vi "autoplace2.vi"(11 "Chain IN":bool) -> (3 "Chain OUT":bool)   [LabVIEW 2010, in "LASA Beta.lvrbt"]
uses:
  LASA Beta.lvrbt
  <vilib>/NXT/NXTIO Xnodes/AddressXNode/NXTIOAddress.xnode
  <vilib>/NXT/Subs/MotorXNode.Servo Type.ctl
  <vilib>/NXT/Subs/MotorXNode.1Servo.ctl
  <vilib>/NXT/Subs/LVHSConnector.ctl
  <vilib>/NXT/NXTIO Xnodes/NXTIOXNode/NXTIO.xnode
  op-run.vi
  <vilib>/NXT/Dual Mode Library/Waits/Wait_Num(msec).vi
  <vilib>/NXT/NXTIO Xnodes/NXTIONodeSubVIs/TETRIX IO Move Servos.vi
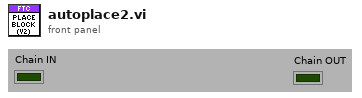
[diagram p1: front panel]
types:
  T1 = typedef "MotorXNode.Servo Type.ctl" = enum16{"Servo"}
  T2 = typedef "LVHSConnector.ctl" = cluster{"Hardware":string, "Flattened String":string}
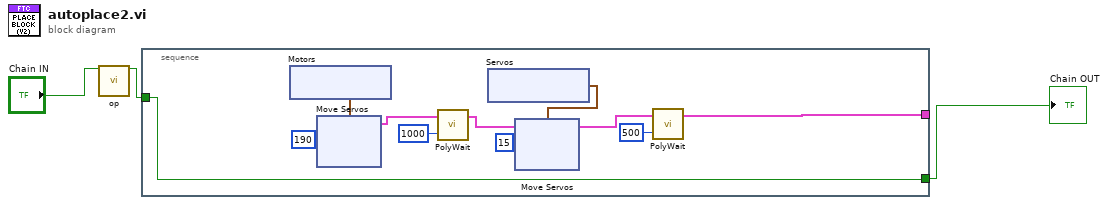
[diagram p0: block diagram]
diagram:
  n1 = call-poly "op.vi"("Chain IN"="Chain IN") -> ("Chain OUT"=w1:bool)  [unwired: 14 in]
  n2 = stacked-sequence {
    tunnel: w1 -> [w4]
    tunnel: [w5] -> _
    tunnel: [w4] -> w3
    frame #0 {
      n3 = xnode "Motors"() -> ("Servo"=w14:cluster{"Servo":T1, "Address":i16})
      n4 = xnode "Move Servos"("Position 1"=u8 190, "Servos"=w14) -> ("NXT"=w11:T2)  [unwired: 1 in]
      n5 = call-poly <vilib>:"PolyWait.vi"("Time (100 msec)"=u32 1000, "NXT"=w11) -> ("NXT"=w8:T2)  [unwired: 2 in]
      n6 = xnode "Servos"() -> ("Servo"=w9:cluster{"Servo":T1, "Address":i16})
      n7 = xnode "Move Servos"("Position 1"=u8 15, "Servos"=w9, "NXT"=w8) -> ("NXT"=w6:T2)
      n8 = call-poly <vilib>:"PolyWait.vi"("Time (100 msec)"=u32 500, "NXT"=w6) -> ("NXT"=w5:T2)  [unwired: 2 in]
    }
  }
  "Chain OUT" <- w3
